vi "StartProcess.vi"(0 "reference in":refnum<class "VCS.lvclass">, 3 "ms timeout (-1)":i32=-1, 5 "Error In":errorcluster) -> (14 "reference out":refnum<class "VCS.lvclass">, 15 "EventFromProcess":refnum<user-event>, 16 "timed out":bool, 19 "Error Out":errorcluster)   [LabVIEW 2023, in "VCS.lvclass"]
doc: "Looks up an existing object matching object name or creates a new object and returns a refnum you can use when calling other class methods.\n\nObjects created with this VI should be destroyed using this class Delete VI."
uses:
  VCS.lvclass
  VCS.lvclass/VCS.ctl
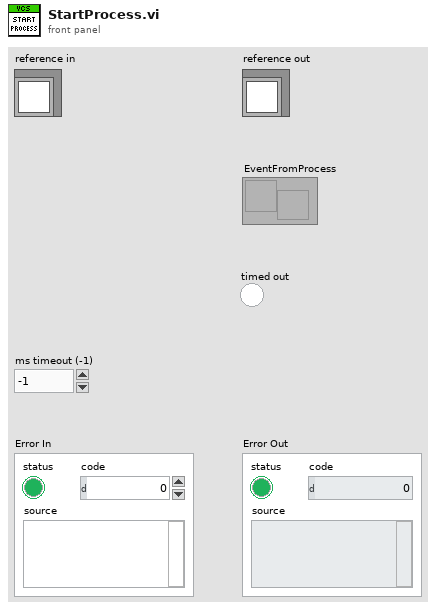
[diagram p1: front panel]
types:
  T1 = enum16{"ReadRepository", "CreateNew", "CreateOrLookUpExisting", "ReadRepositoryAndDestroy"}
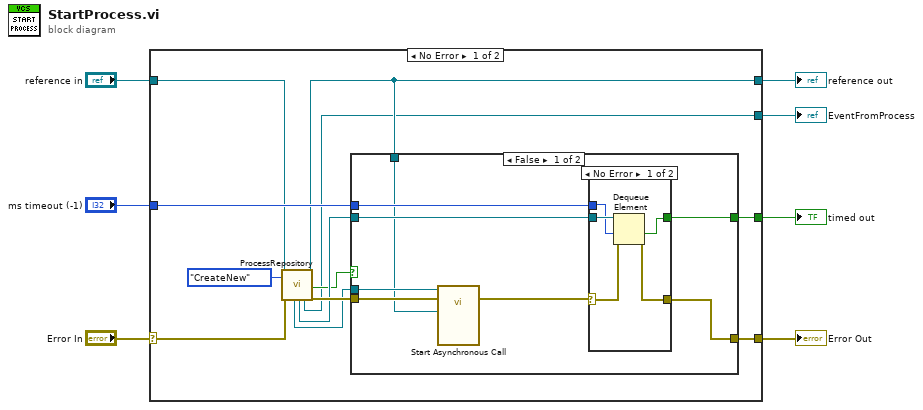
[diagram p0: block diagram]
diagram:
  n1 = case shown="No Error" "Error In" {
    selector: "Error In" -> [w16 w35]
    tunnel: [w17 w35] -> w6
    tunnel: [w12 w36] -> w4
    tunnel: "reference in" -> [w10 w36]
    tunnel: "ms timeout (-1)" -> [w19 _]
    tunnel: [w18 _] -> w2
    tunnel: [w9 _] -> w1
    frame No Error {
      n2 = call "ProcessRepository.vi"("reference in"=w10, "Action(ReadRepository)"=T1."CreateNew", "Error In"=w16) -> ("ProcessViRef"=w14:refnum<vi>, "ProcessSyncQueue"=w13:refnum<queue>, "EventFromProcess"=w9:refnum<user-event>, "reference out"=w12:refnum<class "VCS.lvclass">, "ProcessAlreadyStarted"=w11:bool, "Error Out"=w15:errorcluster)  [unwired: 9 in, 2 out]
      n3 = case shown="False" w11 {
        tunnel: w19 -> [w27 _]
        tunnel: [w26 _] -> w18
        tunnel: [w25 w34] -> w17
        tunnel: w15 -> [w23 w34]
        tunnel: w14 -> [w22 _]
        tunnel: w13 -> [w24 _]
        tunnel: w12 -> [w21 _]
        frame False {
          n4 = call-by-ref "Start Asynchronous Call"(reference=w22, error in=w23, "reference in"=w21) -> (error out=w20:errorcluster)  [unwired: 17 in, 3 out]
          n5 = case shown="No Error" w20 {
            tunnel: w24 -> [w32 _]
            tunnel: w27 -> [w30 _]
            tunnel: [w31 _] -> w26
            selector: w20 -> [w29 w33]
            tunnel: [w28 w33] -> w25
            frame No Error {
              n6 = Dequeue Element(queue=w32, timeout in ms (-1)=w30, error in (no error)=w29) -> (timed out?=w31:bool, error out=w28:errorcluster)  [unwired: 2 out]
            }
            frame Error {
            }
          }
        }
        frame True {
          # "Process Already started.\nThis option will only be used togeather with the\naction: \"CreateOrLookUpExisting\""
        }
      }
    }
    frame Error {
    }
  }
  "Error Out" <- w6
  "reference out" <- w4
  "timed out" <- w2
  "EventFromProcess" <- w1
